vi "FTW-Subscriber-AddAddresses.vi"(0 "FTW-Subscription In":refnum<class "FTW-Subscriber.lvclass">, 5 "Addresses":string, 9 "Connection Timeout":i32=100 format="%d ms", 11 "error in":errorcluster) -> (4 "FTW-Subscription Out":refnum<class "FTW-Subscriber.lvclass">, 15 "error out":errorcluster)   [LabVIEW 2013, in "FTW-Subscriber.lvclass"]
uses:
  FTW-Subscriber.lvclass
  FTW-Subscriber.lvclass/FTW-Subscriber.ctl
  Ether/FTW-Ether-EndpointType.ctl
  Endpoint/FTW-Endpoint.lvclass
  Ether/FTW-Ether.lvclass
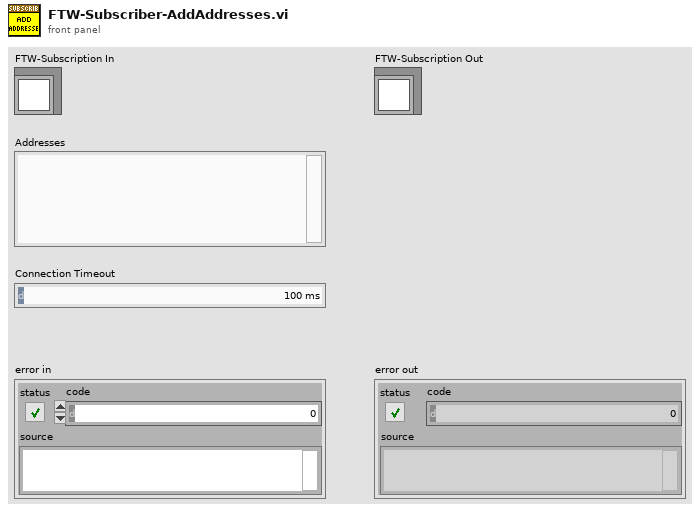
[diagram p1: front panel]
types:
  T1 = typedef "FTW-Ether.lvclass/FTW-Ether-EndpointType.ctl" = enum16{"Server", "Client", "Publisher", "Subscriber"}
  T2 = typedef "FTW-Ether.lvclass/FTW-Ether-MessageTransportScheme.ctl" = enum16{"In process (inproc://)", "TCP (tcp://)"}
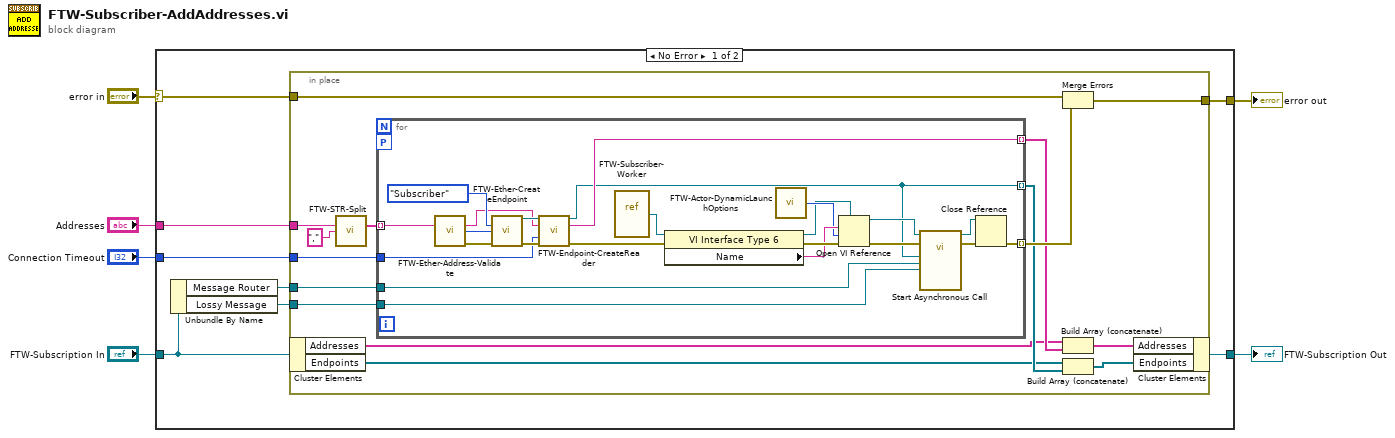
[diagram p0: block diagram]
diagram:
  n1 = case shown="No Error" "error in" {
    selector: "error in" -> [w14 w53]
    tunnel: [w13 w53] -> w2
    tunnel: "Addresses" -> [w12 _]
    tunnel: "FTW-Subscription In" -> [w10 w54]
    tunnel: [w11 w54] -> w4
    tunnel: "Connection Timeout" -> [w7 _]
    frame No Error {
      n2 = Unbundle By Name(w10) -> ("Message Router"=w9:refnum<user-event>, "Lossy Message"=w8:refnum<class "FTW-Message-Lossy.lvclass">)
      n3 = in-place {
        in-place-border: w14 -> [w29]
        in-place-border: [w28] -> w13
        in-place-border: w12 -> [w25]
        in-place-border: w9 -> [w17]
        in-place-border: w8 -> [w16]
        in-place-border: w7 -> [w15]
        n4 = in-place-cluster #1(w10) -> ("Addresses"=w19:string[], "Endpoints"=w18:refnum<class "FTW-Endpoint.lvclass">[])
        n5 = call "FTW-STR-Split.vi"("Delimited String"=w25, "Delimiter"=",") -> ("Array of Strings"=w27:string[])  [unwired: 13 in]
        n6 = for {
          tunnel: [w40] -> w24 mode=indexing
          tunnel: w27 -> [w39] mode=indexing
          tunnel: [w31] -> w22 mode=indexing
          tunnel: [w32] -> w23 mode=indexing
          workers-P: _ -> [_]
          tunnel: w17 -> [w38]
          tunnel: w16 -> [w37]
          tunnel: w15 -> [w30]
          n7 = call "FTW-Ether-Address-Validate.vi"("Address"=w39) -> ("Sanitized Address"=w33:string, "Message Transport Scheme"=w44:T2, "error out"=w42:errorcluster)  [unwired: 12 in]
          n8 = call "FTW-Ether-CreateEndpoint.vi"("Endpoint Type"=FTW-Ether-EndpointType."Subscriber", "Message Transport Scheme"=w44, "error in"=w42) -> ("FTW Endpoint"=w34:refnum<class "FTW-Endpoint.lvclass">, "error out"=w36:errorcluster)  [unwired: 11 in]
          n9 = call-dynamic "FTW-Endpoint-CreateReader.vi"("FTW-Endpoint In"=w34, "Address"=w33, "Connection Timeout"=w30, "error in"=w36) -> ("FTW-Endpoint Out"=w31:refnum<class "FTW-Endpoint.lvclass">, "Actual Address"=w32:string, "error out"=w35:errorcluster)  [unwired: 9 in]
          n10 = vi-ref "FTW-Subscriber-Worker.vi"() -> (w52:refnum<vi>)
          n11 = property class="VI Interface Type 6"(reference=w52, error in=w35) -> (reference out=w48:refnum<vi>, error out=w51:errorcluster, "Name"=w50:string)
          n12 = call "FTW-Actor-DynamicLaunchOptions.vi"() -> ("Open VI Ref Options"=w49:i32)
          n13 = Open VI Reference(type specifier VI Refnum (for type only)=w48, vi path=w50, options=w49, error in (no error)=w51) -> (vi reference=w46:refnum<vi>, error out=w41:errorcluster)  [unwired: 2 in]
          n14 = call-by-ref "Start Asynchronous Call"(reference=w46, error in=w41, "Endpoint"=w31, "Message Handler"=w38, "Lossy Message"=w37) -> (reference out=w45:refnum<vi>, error out=w47:errorcluster)  [unwired: 13 in]
          n15 = Close Reference(reference=w45, error in (no error)=w47) -> (error out=w40:errorcluster)
        }
        n16 = Merge Errors(w29, w24) -> (w28:errorcluster)
        n17 = Build Array (concatenate)(w19, w23) -> (w21:string[])
        n18 = Build Array (concatenate)(w18, w22) -> (w20:refnum<class "FTW-Endpoint.lvclass">[])
        n19 = in-place-cluster #1("Addresses"=w21, "Endpoints"=w20) -> (w11:refnum<class "FTW-Subscriber.lvclass">)
      }
    }
    frame Error {
    }
  }
  "FTW-Subscription Out" <- w4
  "error out" <- w2
